vi "KNNImputer.vi"(8 "error in":errorcluster caption="entrée d'erreur", 11 "KNNImputer":T1={"missing_values"="nan", "n_neighbors"=5, "weights"="uniform", "metric"="nan_euclidean", "copy"=TRUE, "add_indicator"=FALSE}) -> (0 "error out":errorcluster caption="sortie d'erreur", 3 "KNNImputer.lvclass":refnum<class "KNNImputer.lvclass">)   [LabVIEW 2020]
doc: "Imputation for completing missing values using k-Nearest Neighbors.\n\nEach sample’s missing values are imputed using the mean value from n_neighbors nearest neighbors found in the training set. Two samples are close if the features that neither is missing are close.\n\nParameters :\n\n- missing_values : number, string, np.nan or None, default=`np.nan`\n\nThe placeholder for the missing values. All occurrences of missing_values will be imputed. For pandas’ dataframes with nullable integer dtypes with missing values, missing_values should be set to np.nan, since pd.NA will be converted to np.nan.\n\n- n_neighbors : int, default=5\n\nNumber of neighboring samples to use for imputation.\n\n- weights : {‘uniform’, ‘distance’} or callable, default=’uniform’\n\nWeight function used in prediction. Possible values:\n\n‘uniform’ : uniform weights. All points in each neighborhood are weighted equally.\n\n‘distance’ : weight points by the inverse of their distance. in this case, closer neighbors of a query point will have a greater influence than neighbors which are further away.\n\ncallable : a user-defined function which accepts an array of distances, and returns an array of the same shape containing the weights.\n\n- metric : {‘nan_euclidean’} or callable, default=’nan_euclidean’\n\nDistance metric for searching neighbors. Possible values :\n\n‘nan_euclidean’\n\ncallable : a user-defined function.\n\n- copy : bool, default=True\n\nIf True, a copy of X will be created. If False, imputation will be done in-place whenever possible.\n\n- add_indicator : bool, default=False\n\nIf True, a MissingIndicator transform will stack onto the output of the imputer’s transform. This allows a predictive estimator to account for missingness despite imputation. If a feature has no missing values at fit/train time, the feature won’t appear on the missing indicator even if there are missing values at transform/test time.\n\n\nMethods : \n\n- Fit :\n\nFit the imputer on X.\n\nParameters : X : array-like shape of (n_samples, n_features)\n Input data, where n_samples is the number of samples and n_features is the number of features.\n\n\n- Fit Transform : \n\nFit to data, then transform it.\n\nFits transformer to X and y with optional parameters fit_params and returns a transformed version of X.\n\nParameters : X : {array-like, sparse matrix, dataframe} of shape (n_samples, n_features)\n y : ndarray of shape (n_samples,), default=None\n Target values.\n\nReturns : X_new : ndarray array of shape (n_samples, n_features_new)\n Transformed array.\n\n\n- Transform : \n\nImpute all missing values in X.\n\nParameters : X : array-like of shape (n_samples, n_features)\n The input data to complete.\n\nReturns : X : array-like of shape (n_samples, n_output_features)\n The imputed dataset. n_output_features is the number of features that is not always missing during fit."
uses:
  KNNImputer.lvclass
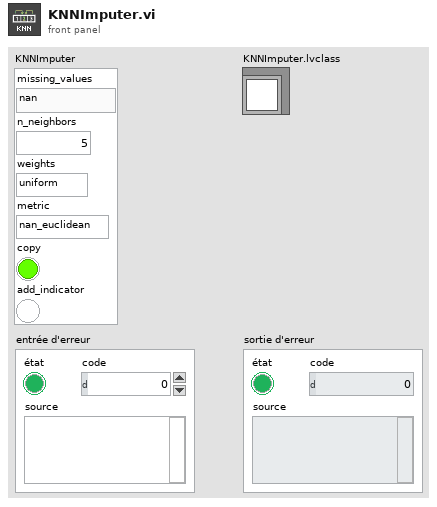
[diagram p1: front panel]
types:
  T1 = cluster{"missing_values":string, "n_neighbors":i32, "weights":string, "metric":string, "copy":bool, "add_indicator":bool}
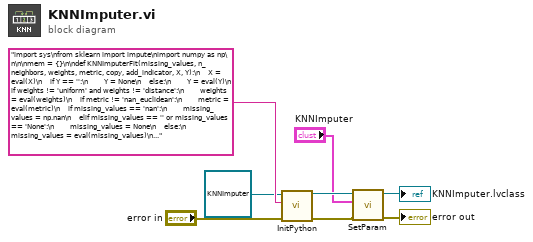
[diagram p0: block diagram]
diagram:
  n1 = call-dynamic "InitPython.vi"("error in (no error)"="error in", "Python Instruction"="import sys\nfrom sklearn import impute\nimport numpy as np\n\n\nmem = {}\n\ndef KNNImputerFit(missing_values, n_neighbors, weights, metric, copy, add_indicator, X, Y):\n    X = eval(X)\n    if Y == '':\n        Y = None\n    else:\n        Y = eval(Y)\n    if weights != 'uniform' and weights != 'distance':\n        weights = eval(weights)\n    if metric != 'nan_euclidean':\n        metric = eval(metric)\n    if missing_values == 'nan':\n        missing_values = np.nan\n    elif missing_values == '' or missing_values == 'None':\n        missing_values = None\n    else:\n        missing_values = eval(missing_values)\n    try:\n        KNNImputer = impute.KNNImputer(missing_values, n_neighbors, weights, metric, copy, add_indicator).fit(X, Y)\n        mem['FitKNNImputer'] = KNNImputer\n        return str('OK')\n    except:\n        erreur = sys.exc_info()\n        typerr = u\"%s\" % (erreur[0])\n        typerr = typerr[typerr.find(\"'\")+1:typerr.rfind(\"'\")]\n        msgerr = u\"%s\" % (erreur[1])\n        message = str('/!\\\\ {0} : {1}'. format(typerr,msgerr))\n        return message \n\ndef KNNImputerFitTransform(missing_values, n_neighbors, weights, metric, copy, add_indicator, X, Y):\n    X = eval(X)\n    if Y == '':\n        Y = None\n    else:\n        Y = eval(Y)\n    if weights != 'uniform' and weights != 'distance':\n        weights = eval(weights)\n    if metric != 'nan_euclidean':\n        metric = eval(metric)\n    if missing_values == 'nan':\n        missing_values = np.nan\n    elif missing_values == '' or missing_values == 'None':\n        missing_values = None\n    else:\n        missing_values = eval(missing_values)\n    try:\n        KNNImputer = impute.KNNImputer(missing_values, n_neighbors, weights, metric, copy, add_indicator).fit_transform(X, Y)\n        KNNImputer = KNNImputer.tolist()\n        return str(KNNImputer)\n    except:\n        erreur = sys.exc_info()\n        typerr = u\"%s\" % (erreur[0])\n        typerr = typerr[typerr.find(\"'\")+1:typerr.rfind(\"'\")]\n        msgerr = u\"%s\" % (erreur[1])\n        message = str('/!\\\\ {0} : {1}'. format(typerr,msgerr))\n        return message \n    \n\ndef KNNImputerTransform(missing_values, n_neighbors, weights, metric, copy, add_indicator, X, Y):  \n    X = eval(X)\n    if Y == '':\n        Y = None\n    else:\n        Y = eval(Y)\n    if weights != 'uniform' and weights != 'distance':\n        weights = eval(weights)\n    if metric != 'nan_euclidean':\n        metric = eval(metric)\n    if missing_values == 'nan':\n        missing_values = np.nan\n    elif missing_values == '' or missing_values == 'None':\n        missing_values = None\n    else:\n        missing_values = eval(missing_values)\n    try:\n        KNNImputer = mem['FitKNNImputer'].transform(X, Y)\n        KNNImputer = KNNImputer.tolist()\n        return str(KNNImputer)\n    except:\n        erreur = sys.exc_info()\n        typerr = u\"%s\" % (erreur[0])\n        typerr = typerr[typerr.find(\"'\")+1:typerr.rfind(\"'\")]\n        msgerr = u\"%s\" % (erreur[1])\n        message = str('/!\\\\ {0} : {1}'. format(typerr,msgerr))\n        return message", "Scikit-learn en entrée"=refnum<class "KNNImputer.lvclass"> refnum ("KNNImputer.lvclass")) -> ("error out"=w5:errorcluster, "Scikit-learn en sortie"=w4:refnum<class "KNNImputer.lvclass">)  [unwired: 7 in]
  n2 = call-dynamic "SetParam.vi"("error in (no error)"=w5, "KNNImputer"="KNNImputer", "KNNImputer.lvclass"=w4) -> ("error out"=→"error out":errorcluster, "KNNImputer.lvclass"=→"KNNImputer.lvclass":refnum<class "KNNImputer.lvclass">)  [unwired: 7 in]
